vi "Connection POC.vi"() -> ()   [LabVIEW 2013]
uses:
  <vilib>/httpClient/ClientHandle.ctl
  <vilib>/httpClient/LabVIEWHTTPClient.lvlib
panel:
  in  "Stop Button":bool
  out "body":string
  out "headers":string
  out "error out":errorcluster
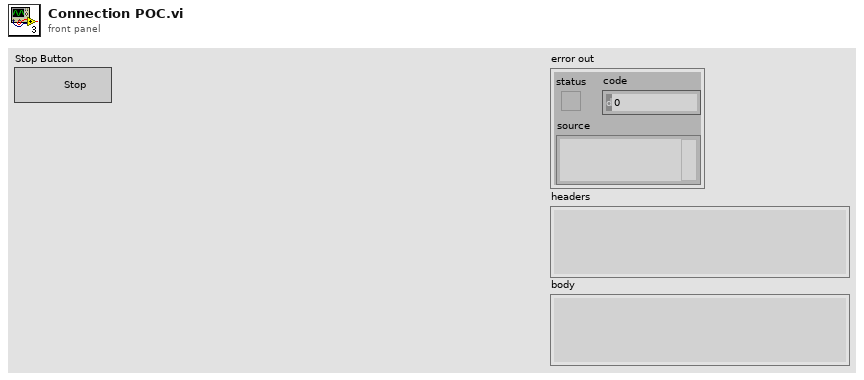
[diagram p1: front panel]
types:
  T1 = typedef "LabVIEWHTTPClient.lvlib/ClientHandle.ctl" = refnum<k1>
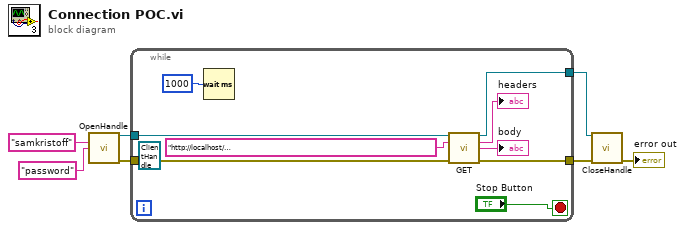
[diagram p0: block diagram]
diagram:
  n1 = call <vilib>:"OpenHandle.vi"("username"="samkristoff", "password"="password" ("username")) -> ("client handle out"=w7:T1, "error out"=w6:errorcluster)  [unwired: 12 in]
  n2 = while {
    tunnel: w7 -> [w16]
    tunnel: w6 -> [w15]
    tunnel: [w13] -> w5
    tunnel: [w12] -> w4
    stop <- "Stop Button" stop-if-true
    (unwired) T1 refnum ("client handle out")
    n3 = Wait (ms)(milliseconds to wait=u32 1000) -> ()  [unwired: 1 out]
    n4 = call <vilib>:"GET.vi"("client handle"=w16, "url"="http://localhost/jsonrpc?request={%22jsonrpc%22:%222.0%22,%22method%22:%22Input.ExecuteAction%22,%22params%22:{%22action%22:%22left%22},%22id%22:1}", "error in (no error)"=w15) -> ("client handle out"=w13:T1, "headers"=→"headers":string, "body"=→"body":string, "error out"=w12:errorcluster)  [unwired: 9 in]
  }
  n5 = call <vilib>:"CloseHandle.vi"("client handle"=w5, "error in (no error)"=w4) -> ("error out"=→"error out":errorcluster)  [unwired: 13 in]
